vi "DAQ - 1 Module - SubVI.vi"(11 "array":dbl[](array[numeric])) -> (3 "output array":dbl[](array[numeric]))   [LabVIEW 2013]
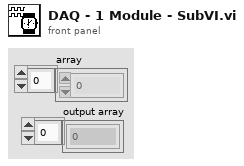
[diagram p1: front panel]
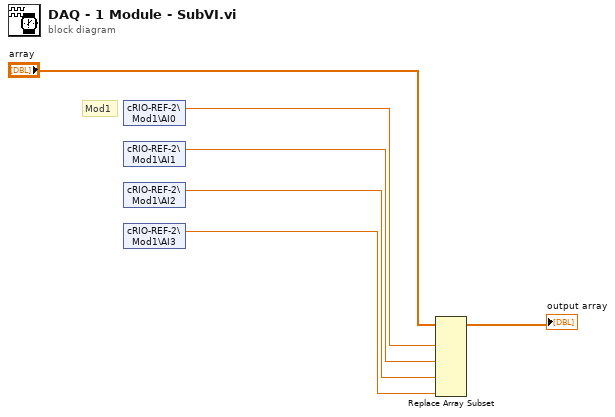
[diagram p0: block diagram]
diagram:
  # "Mod1"
  n1 = shared-variable "cRIO-REF-2\\Mod1\\AI0"() -> (w6:dbl)  [unwired: 1 in, 1 out]
  n2 = shared-variable "cRIO-REF-2\\Mod1\\AI1"() -> (w5:dbl)  [unwired: 1 in, 1 out]
  n3 = shared-variable "cRIO-REF-2\\Mod1\\AI2"() -> (w4:dbl)  [unwired: 1 in, 1 out]
  n4 = shared-variable "cRIO-REF-2\\Mod1\\AI3"() -> (w3:dbl)  [unwired: 1 in, 1 out]
  n5 = Replace Array Subset(array="array", new element #1=w6, new element #2=w5, new element #3=w4, new element #4=w3) -> (→"output array":dbl[])  [unwired: 4 in]
